vi "SetWaveformParameters.vi"(8 "error in (no error)":errorcluster, 10 "Waveform Parameters":T1={"Duty Cycle"=50.0, "Frequency"=1000.0, "Waveform Function"=0, "Amplitude"=2.0, "DC Offset"=0.0} {"Waveform Function" items=["Sine", "Square", "Triangle/Ramp", "DC"]}, 11 "OutputWaveform in":refnum<class "OutputWaveform.lvclass">) -> (0 "error out":errorcluster, 3 "OutputWaveform out":refnum<class "OutputWaveform.lvclass">)   [LabVIEW 2020, in "OutputWaveform.lvclass"]
uses:
  OutputWaveform.lvclass
  OutputWaveform.lvclass/OutputWaveform.ctl
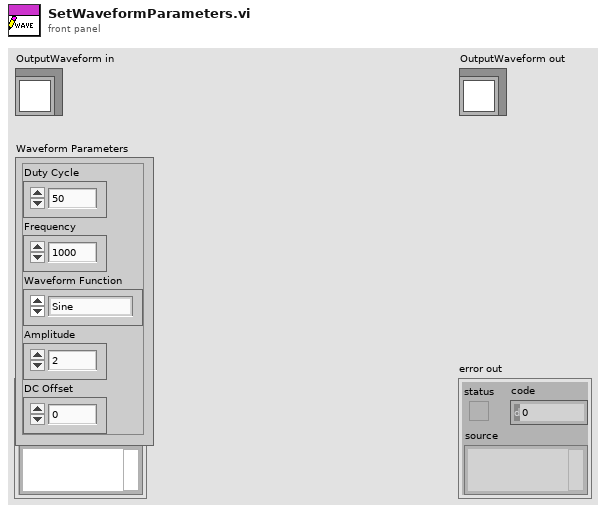
[diagram p1: front panel]
types:
  T1 = cluster{"Duty Cycle":dbl, "Frequency":dbl, "Waveform Function":i32, "Amplitude":dbl, "DC Offset":dbl}
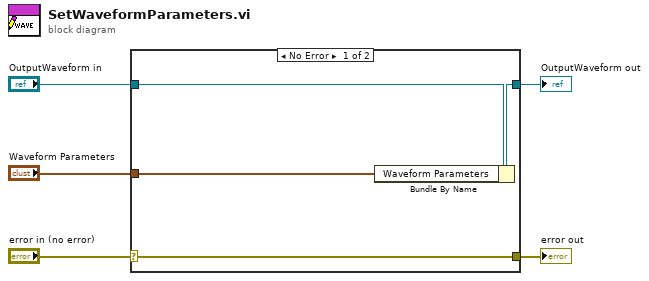
[diagram p0: block diagram]
diagram:
  n1 = case shown="No Error" "error in (no error)" {
    selector: "error in (no error)" -> [w9 w10]
    tunnel: [w9 w10] -> w4
    tunnel: [w7 w11] -> w2
    tunnel: "OutputWaveform in" -> [w8 w11]
    tunnel: "Waveform Parameters" -> [w6 _]
    frame No Error {
      n2 = Bundle By Name(cluster=w8, "Waveform Parameters"=w6) -> (w7:refnum<class "OutputWaveform.lvclass">)
    }
    frame Error {
    }
  }
  "error out" <- w4
  "OutputWaveform out" <- w2
